vi "dllshutdown.vi"() -> (3 "function return":i32)   [LabVIEW 2013, in "C37118-DLL.lvlib" / "StrongridDLL.lvlib"]
doc: "STRONGRIDIEEEC37118DLL_API int __cdecl dllshutdown();"
uses:
  StrongridDLL.lvlib
  builds/StrongridDLL/StrongridDLL.dll
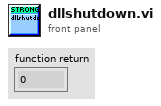
[diagram p1: front panel]
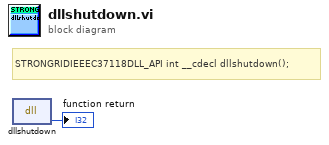
[diagram p0: block diagram]
diagram:
  # "STRONGRIDIEEEC37118DLL_API int __cdecl dllshutdown();"
  n1 = dll-call lib="C:/dev/OSS/S3DK/builds/StrongridDLL/StrongridDLL.*" fn="dllshutdown"() -> (→"function return":i32)  [unwired: 3 in, 2 out]
